vi "Actor Core.vi"(8 "error in":errorcluster, 11 "Assert Startup UI in":refnum<class "Assert Startup UI.lvclass">) -> (0 "error out":errorcluster, 3 "Actor out":refnum<class "Actor.lvclass">)   [LabVIEW 2016, in "Assert API Components.lvlib" / "Assert Startup UI.lvlib" / "Assert Startup UI.lvclass"]
doc: "(<B>Filename</B>: Actor Framework.lvlib:Actor.lvclass:Actor Core.vi)\n\nReceives messages to the actor, reacts to them, and initiates any error handling that may shut the actor down.\n\nDescendant classes may override this VI to append parallel tasks for the actor to complete while it handles messages. Overrides use the Call Parent Method node."
uses:
  Assert Startup UI.lvclass
  C:/Program Files (x86)/National Instruments/LabVIEW 2016/vi.lib/ActorFramework/Actor/Actor.lvclass
  C:/Users/ukhornp/Documents/Assert API/Core/Base UI Actor/Base UI Actor/Base UI Actor.lvclass
  <vilib>/ActorFramework/Actor/Actor.lvclass
  Base UI Actor/Base UI Actor/Base UI Actor.lvclass/Base UI Actor.ctl
  <vilib>/ActorFramework/Actor/Actor.lvclass/Actor.ctl
  <vilib>/ActorFramework/Message Enqueuer/Message Enqueuer.lvclass/Message Enqueuer.ctl
  Assert API Components/Display Type.ctl
  Assert Startup UI Messages/Launch New Display Msg/Launch New Display Msg.lvclass/Launch New Display Msg.ctl
  <vilib>/ActorFramework/Message Enqueuer/Init from Existing Queue.vi
  <vilib>/ActorFramework/Message Enqueuer/Enqueue.vi
  <vilib>/ActorFramework/Stop Msg/Stop Msg.lvclass
  C:/Program Files (x86)/National Instruments/LabVIEW 2016/vi.lib/ActorFramework/Message/Message.lvclass
  Assert Startup UI Messages/Launch New Display Msg/Launch New Display Msg.lvclass
  <vilib>/Utility/LVClass/Get LV Class Name.vi
  <resource>/AFDebug/Generate Trace for Message.vi
  <vilib>/ActorFramework/Message Priority Queue/Priority Enqueue.vi
  Base UI Actor/Base UI Actor/Base UI Actor.lvclass
  <vilib>/ActorFramework/Message Enqueuer/Message Enqueuer.lvclass
  Assert API Components/Assert API Components.lvlib
panel:
  in  "Add Display":bool
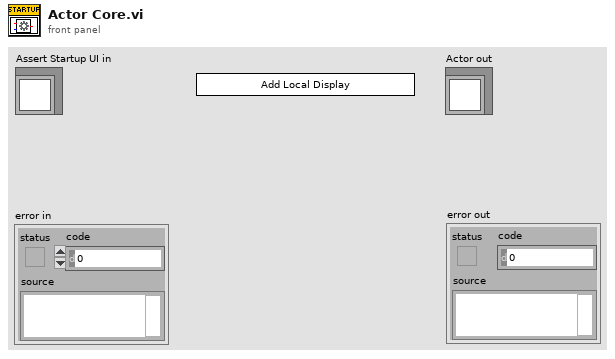
[diagram p1: front panel]
types:
  T1 = enum32{"Invalid", "Standard", "Closed", "Hidden", "Minimized", "Maximized"}
  T2 = typedef "Assert API Components.lvlib/Display Type.ctl" = enum16{"Local", "Network"}
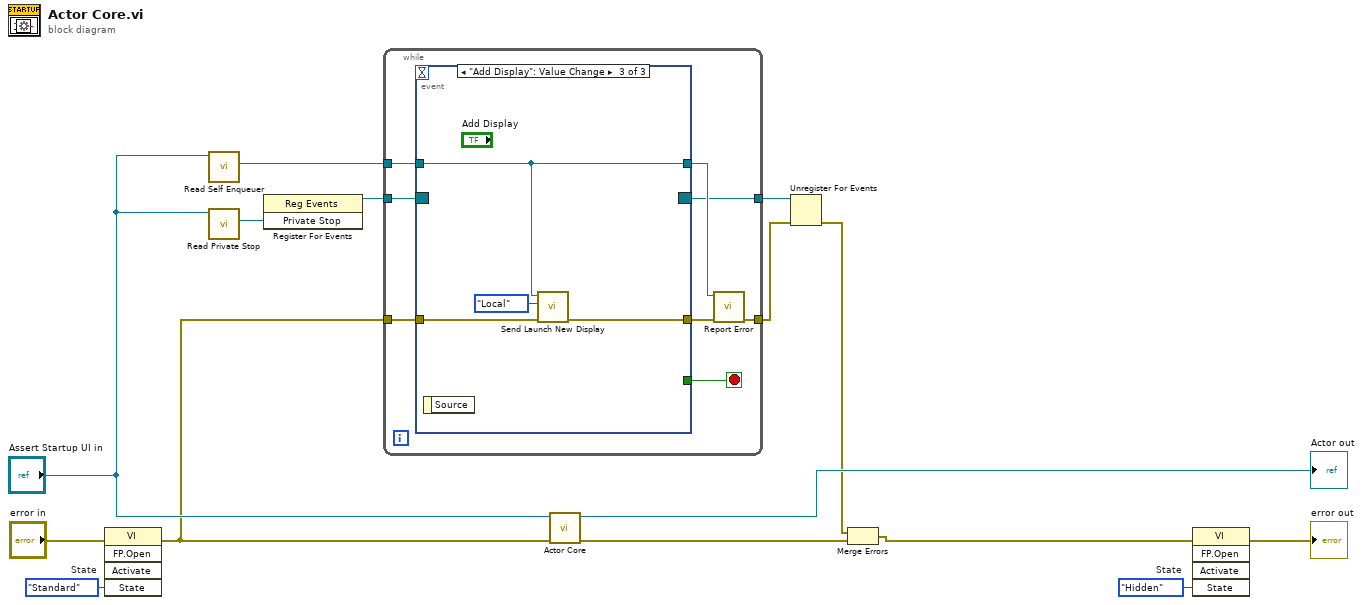
[diagram p0: block diagram]
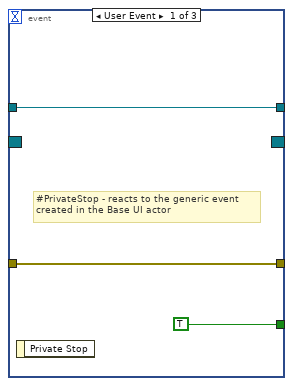
[diagram p2: hidden frame]
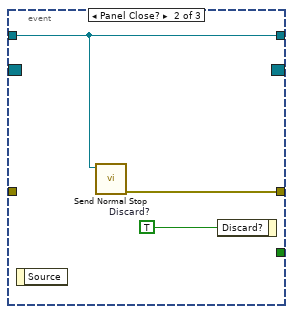
[diagram p3: hidden frame]
diagram:
  w2 = T1."Standard"  # State
  w3 = T1."Hidden"  # State
  n1 = invoke class="VI" method="FP.Open"(error in="error in", "State"=w2) -> (error out=w1:errorcluster)  [unwired: 3 in, 4 out]
  n2 = call <vilib>:"Read Self Enqueuer.vi"("Actor"="Assert Startup UI in") -> ("Self Enqueuer"=w9:refnum<class "Message Enqueuer.lvclass">)  [unwired: 10 in]
  n3 = call "Read Private Stop.vi"("Base UI Actor in"="Assert Startup UI in") -> ("Private Stop"=w13:refnum<user-event>)  [unwired: 10 in]
  n4 = register-events(w13) -> (reference out=w12:refnum<event-registration>)  [unwired: 2 in, 1 out]
  n5 = while {
    tunnel: w12 -> [w23]
    tunnel: w9 -> [w21]
    tunnel: w1 -> [w20]
    tunnel: [w18] -> w6
    tunnel: [w16] -> w7
    stop <- w22 stop-if-true
    n6 = event shown="[2] \"Add Display\": Value Change" {
      selector: w23 -> [_ _ _]
      dyn-events: [_ _ _] -> w16
      timeout: _ -> [_ _ _]
      tunnel: [TRUE _ _] -> w22
      tunnel: w21 -> [w24 w28 w31]
      tunnel: w20 -> [w25 _ w33]
      tunnel: [w24 w28 w31] -> w17
      tunnel: [w25 w27 w32] -> w19
      event User Event {
        # "#PrivateStop - reacts to the generic event created in the Base UI actor"
        n7 = event-data() -> ()  [unwired: 1 in, 1 out]
      }
      event Panel Close? {
        w29 = TRUE  # Discard?
        n8 = event-data() -> ()  [unwired: 1 in, 1 out]
        n9 = call <vilib>:"Send Normal Stop.vi"("Message Enqueuer"=w28) -> ("error out"=w27:errorcluster)  [unwired: 10 in]
        n10 = event-data("Discard?"=w29) -> ()  [unwired: 1 in, 1 out]
      }
      event "Add Display": Value Change {
        n11 = event-data() -> ()  [unwired: 1 in, 1 out]
        n12 = call "Send Launch New Display.vi"("error in (no error)"=w33, "Display Type"=Display_Type."Local", "Message Enqueuer"=w31) -> ("error out"=w32:errorcluster)  [unwired: 7 in, 1 out]
      }
    }
    n13 = call "Report Error.vi"("error in (no error)"=w19, "Self Enqueuer"=w17) -> ("error out"=w18:errorcluster)  [unwired: 9 in]
  }
  n14 = call-parent "Actor Core.vi"("error in"=w1, "Actor in"="Assert Startup UI in") -> ("error out"=w15:errorcluster, "Actor out"=→"Actor out":refnum<class "Actor.lvclass">)  [unwired: 8 in]
  n15 = Unregister For Events(event registration refnum=w7, error in=w6) -> (error out=w5:errorcluster)
  n16 = Merge Errors(w5, w15) -> (w8:errorcluster)
  n17 = invoke class="VI" method="FP.Open"(error in=w8, "State"=w3) -> (error out=→"error out":errorcluster)  [unwired: 3 in, 4 out]
